vi "EditItem__slk_tc.vi"(0 "tree control in":refnum<class "TreeControl.lvclass">, 1 "symbol (no change=-1)":i32, 5 "input tag (current tag)":string, 7 "new tag (no change)":string, 9 "new text":string, 11 "error in (no error)":errorcluster, 12 "column # (0)":i32) -> (4 "tree control out":refnum<class "TreeControl.lvclass">, 15 "error out":errorcluster)   [LabVIEW 2020, in "TreeControl.lvclass"]
doc: "Modifies item from tree. Uses the current selection if there is no item input. If there is no item selected within the tree it modifies nothing."
uses:
  Library/TreeControl.lvclass
  Library/TreeControl.lvclass/TreeControl.ctl
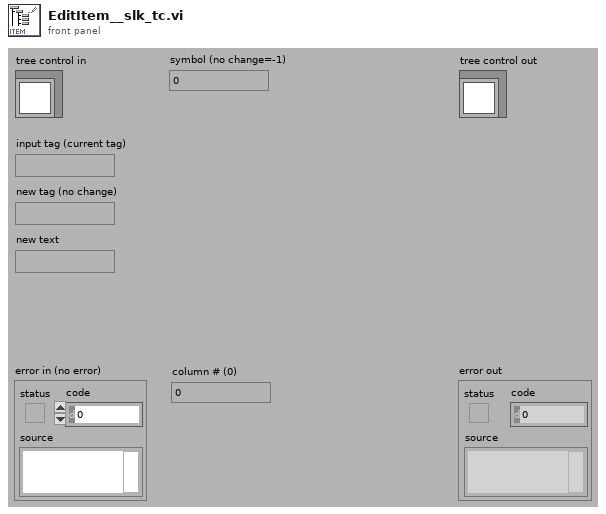
[diagram p1: front panel]
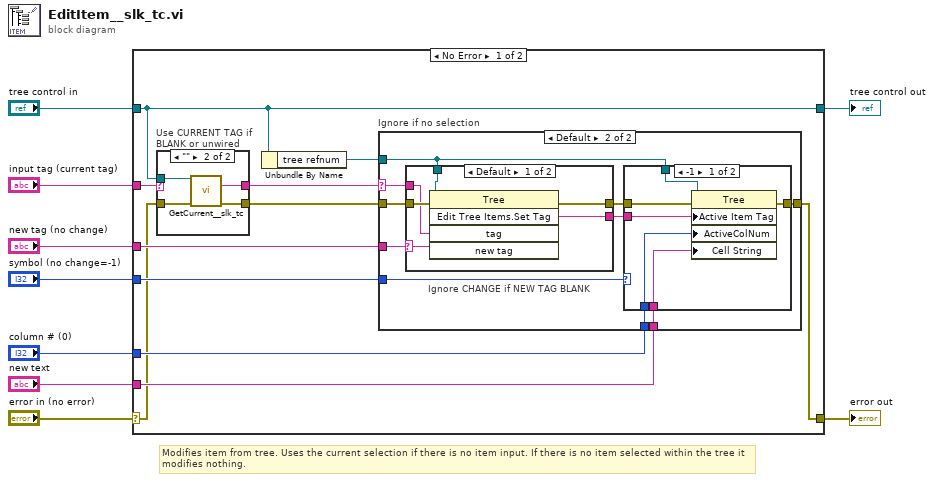
[diagram p0: block diagram]
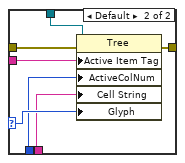
[diagram p3: hidden frame]
diagram:
  # "Modifies item from tree. Uses the current selection if there is no item input. If there is no item selected within the tree it modifies nothing."
  n1 = case shown="No Error" "error in (no error)" {
    selector: "error in (no error)" -> [w11 w60]
    tunnel: [w10 w60] -> w8
    tunnel: [w18 w59] -> w6
    tunnel: "tree control in" -> [w18 w59]
    tunnel: "input tag (current tag)" -> [w20 _]
    tunnel: "new tag (no change)" -> [w15 _]
    tunnel: "symbol (no change=-1)" -> [w14 _]
    tunnel: "column # (0)" -> [w13 _]
    tunnel: "new text" -> [w12 _]
    frame No Error {
      n2 = case "Use CURRENT TAG if BLANK or unwired" shown="\"\"" w20 {
        selector: w20 -> [w54 _]
        tunnel: [w54 w58] -> w16
        tunnel: w18 -> [_ w57]
        tunnel: w11 -> [w53 w56]
        tunnel: [w53 w55] -> w19
        frame Default {
        }
        frame "" {
          n3 = call "GetCurrent__slk_tc.vi"("tree control in"=w57, "error in (no error)"=w56) -> ("current tag"=w58:string, "error out"=w55:errorcluster)  [unwired: 1 in, 11 out]
        }
      }
      n4 = Unbundle By Name(w18) -> ("tree refnum"=w17:refnum<vi>)
      n5 = case "Ignore if no selection" shown="Default" w16 {
        selector: w16 -> [_ w30]
        tunnel: w19 -> [w21 w29]
        tunnel: w17 -> [_ w28]
        tunnel: w15 -> [_ w31]
        tunnel: w14 -> [_ w27]
        tunnel: w13 -> [_ w24]
        tunnel: w12 -> [_ w23]
        tunnel: [w21 w22] -> w10
        frame "" {
        }
        frame Default {
          n6 = case "Ignore CHANGE if NEW TAG BLANK" shown="Default" w31 {
            selector: w31 -> [w50 _]
            tunnel: w30 -> [w47 w51]
            tunnel: w29 -> [w49 w52]
            tunnel: [w48 w52] -> w25
            tunnel: [w46 w51] -> w26
            tunnel: w28 -> [w45 _]
            frame Default {
              n7 = invoke class="Tree" method="Edit Tree Items.Set Tag"(reference=w45, error in=w49, "tag"=w47, "new tag"=w50) -> (error out=w48:errorcluster, "Edit Tree Items:Set Tag"=w46:string)  [unwired: 1 in, 3 out]
            }
            frame "" {
            }
          }
          n8 = case shown="-1" w27 {
            selector: w27 -> [_ w40]
            tunnel: w28 -> [w37 w44]
            tunnel: w26 -> [w36 w43]
            tunnel: w25 -> [w35 w42]
            tunnel: [w34 w41] -> w22
            tunnel: w24 -> [w33 w39]
            tunnel: w23 -> [w32 w38]
            frame -1 {
              n9 = property class="Tree"(reference=w37, error in=w35, "Active Item Tag"=w36, "ActiveColNum"=w33, "Cell String"=w32) -> (error out=w34:errorcluster)  [unwired: 1 out]
            }
            frame Default {
              n10 = property class="Tree"(reference=w44, error in=w42, "Active Item Tag"=w43, "ActiveColNum"=w39, "Cell String"=w38, "Glyph"=w40) -> (error out=w41:errorcluster)  [unwired: 1 out]
            }
          }
        }
      }
    }
    frame Error {
    }
  }
  "error out" <- w8
  "tree control out" <- w6
